vi "SetBeverage.lvclass.vi"(8 "error in (no error)":errorcluster, 10 "Beverage.lvclass":refnum<class "Beverage.lvclass">, 11 "object in":refnum<class "CondimentDecorator.lvclass">) -> (0 "error out":errorcluster, 3 "object out":refnum<class "CondimentDecorator.lvclass">)   [LabVIEW 2021, in "CondimentDecorator.lvclass"]
uses:
  CondimentDecorator.lvclass
  CondimentDecorator.lvclass/CondimentDecorator.ctl
  Beverage/Beverage.lvclass
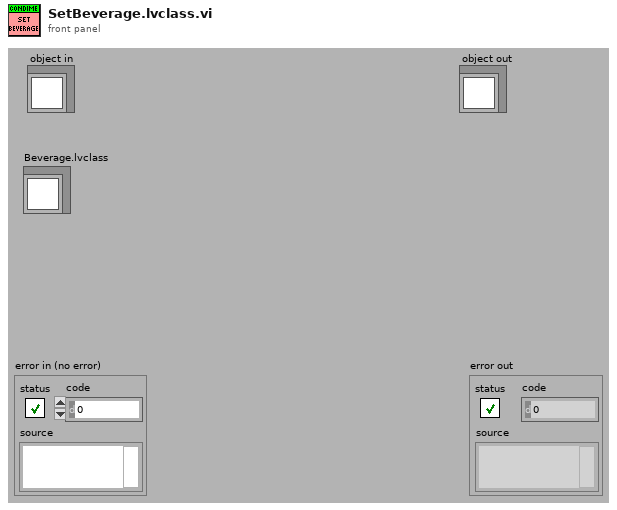
[diagram p1: front panel]
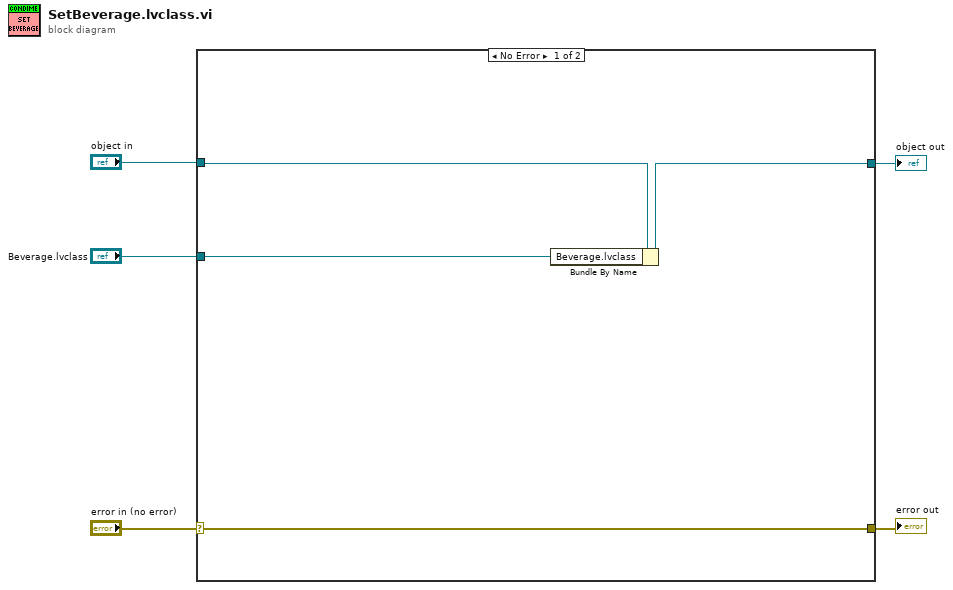
[diagram p0: block diagram]
diagram:
  n1 = case shown="No Error" "error in (no error)" {
    selector: "error in (no error)" -> [w8 w11]
    tunnel: [w8 w11] -> w4
    tunnel: [w6 w10] -> w2
    tunnel: "object in" -> [w7 w10]
    tunnel: "Beverage.lvclass" -> [w9 _]
    frame No Error {
      n2 = Bundle By Name(cluster=w7, "Beverage.lvclass"=w9) -> (w6:refnum<class "CondimentDecorator.lvclass">)
    }
    frame Error {
    }
  }
  "error out" <- w4
  "object out" <- w2
